vi "new FGGA Serial Data Server & Recordingv4.3_10Hz.vi"(0 "VISA resource name out":refnum<visa-resource-name>, 11 "error IO":errorcluster) -> ()   [LabVIEW 2014]
uses:
  <vilib>/Platform/TimedLoop/XDataNode/timing_clust.ctl
  <vilib>/Platform/TimedLoop/XDataNode/nitl_modes.ctl
  <vilib>/Platform/TimedLoop/XDataNode/wakeup.ctl
  C:/Program Files (x86)/National Instruments/LabVIEW 2014/examples/Data Communication/Network Streams/Simple Network Streams/support/Network Stream Command.ctl
  <vilib>/Utility/error.llb/whitespace.ctl
  <vilib>/Instr/_visa.llb/VISA Flush IO Buffer Mask.ctl
  <vilib>/Instr/_visa.llb/VISA Configure Serial Port (Instr).vi
  <vilib>/Utility/tcp.llb/UDP Multicast Write-Only Open.vi
  <vilib>/platform/TimedLoop/XDataNode/XDataNode.xnode
  <vilib>/Platform/TimedLoop/XDataNode/XDNodeRunTimeDep.lvlib
panel:
  out "ASCII_file_out":string
  out "Unix time":u32
  out "FGGA Pump":bool
  out "Flight Number":string
  out "Stop File Write":bool
  out "Default file name":string
  out "MFC":dbl[](array[numeric])
  out "FGGA restart":bool
  out "V4":bool
  out "V3":bool
  out "V2":bool
  out "V1":bool
  out "error out 2":errorcluster
  out "error out":errorcluster
  in  "MFC_1 SLPM set value":dbl
  out "Value Read":string
  out "status":bool
  in  "VISA resource name":refnum<visa-resource-name>="ASRL3::INSTR"
  in  "timeout (10sec) 2":u32=3000
  in  "Clear Display\nErrors":bool
  out "Data Processing":bool
  out "TCP Binary Packet":string
  out "UDP Time Stamp Offset":i32=1
  out "Data String":string
  out "UDP_ACSII_Out":string
  out "Serial error out":errorcluster
  out "SEPTIC TCP Error Out":errorcluster
  out "TCP packet\nSend To SEPTIC":bool
  out "FISH TCP Error Out":errorcluster
  out "TCP packet\nSend To FISH":bool
  out "UDP_Pack_num":u32
  out "UDP_Out Status":bool
  out "UDP_Out_Error Out":errorcluster
  out "Data Array":string[](array[string])
  out "RAW DATA":string
  in  "stop":bool
  out "Number of times \nRead time out":u32
  out "Loop count":i32
  # "Date"
  # "Time"
  # "CH4_wet_ppm"
  # "1"
  # "H2O_ppm"
  # "CO2_wet_ppm"
  # "CH4_dry_ppm"
  # "CO2_dry_ppm"
  # "cell_pressure_torr"
  # "cell_temp_degC"
  # "ambient(bench)_temp_degC"
  # "RDA_us"
  # "RDB_us"
  # "Fitflag"
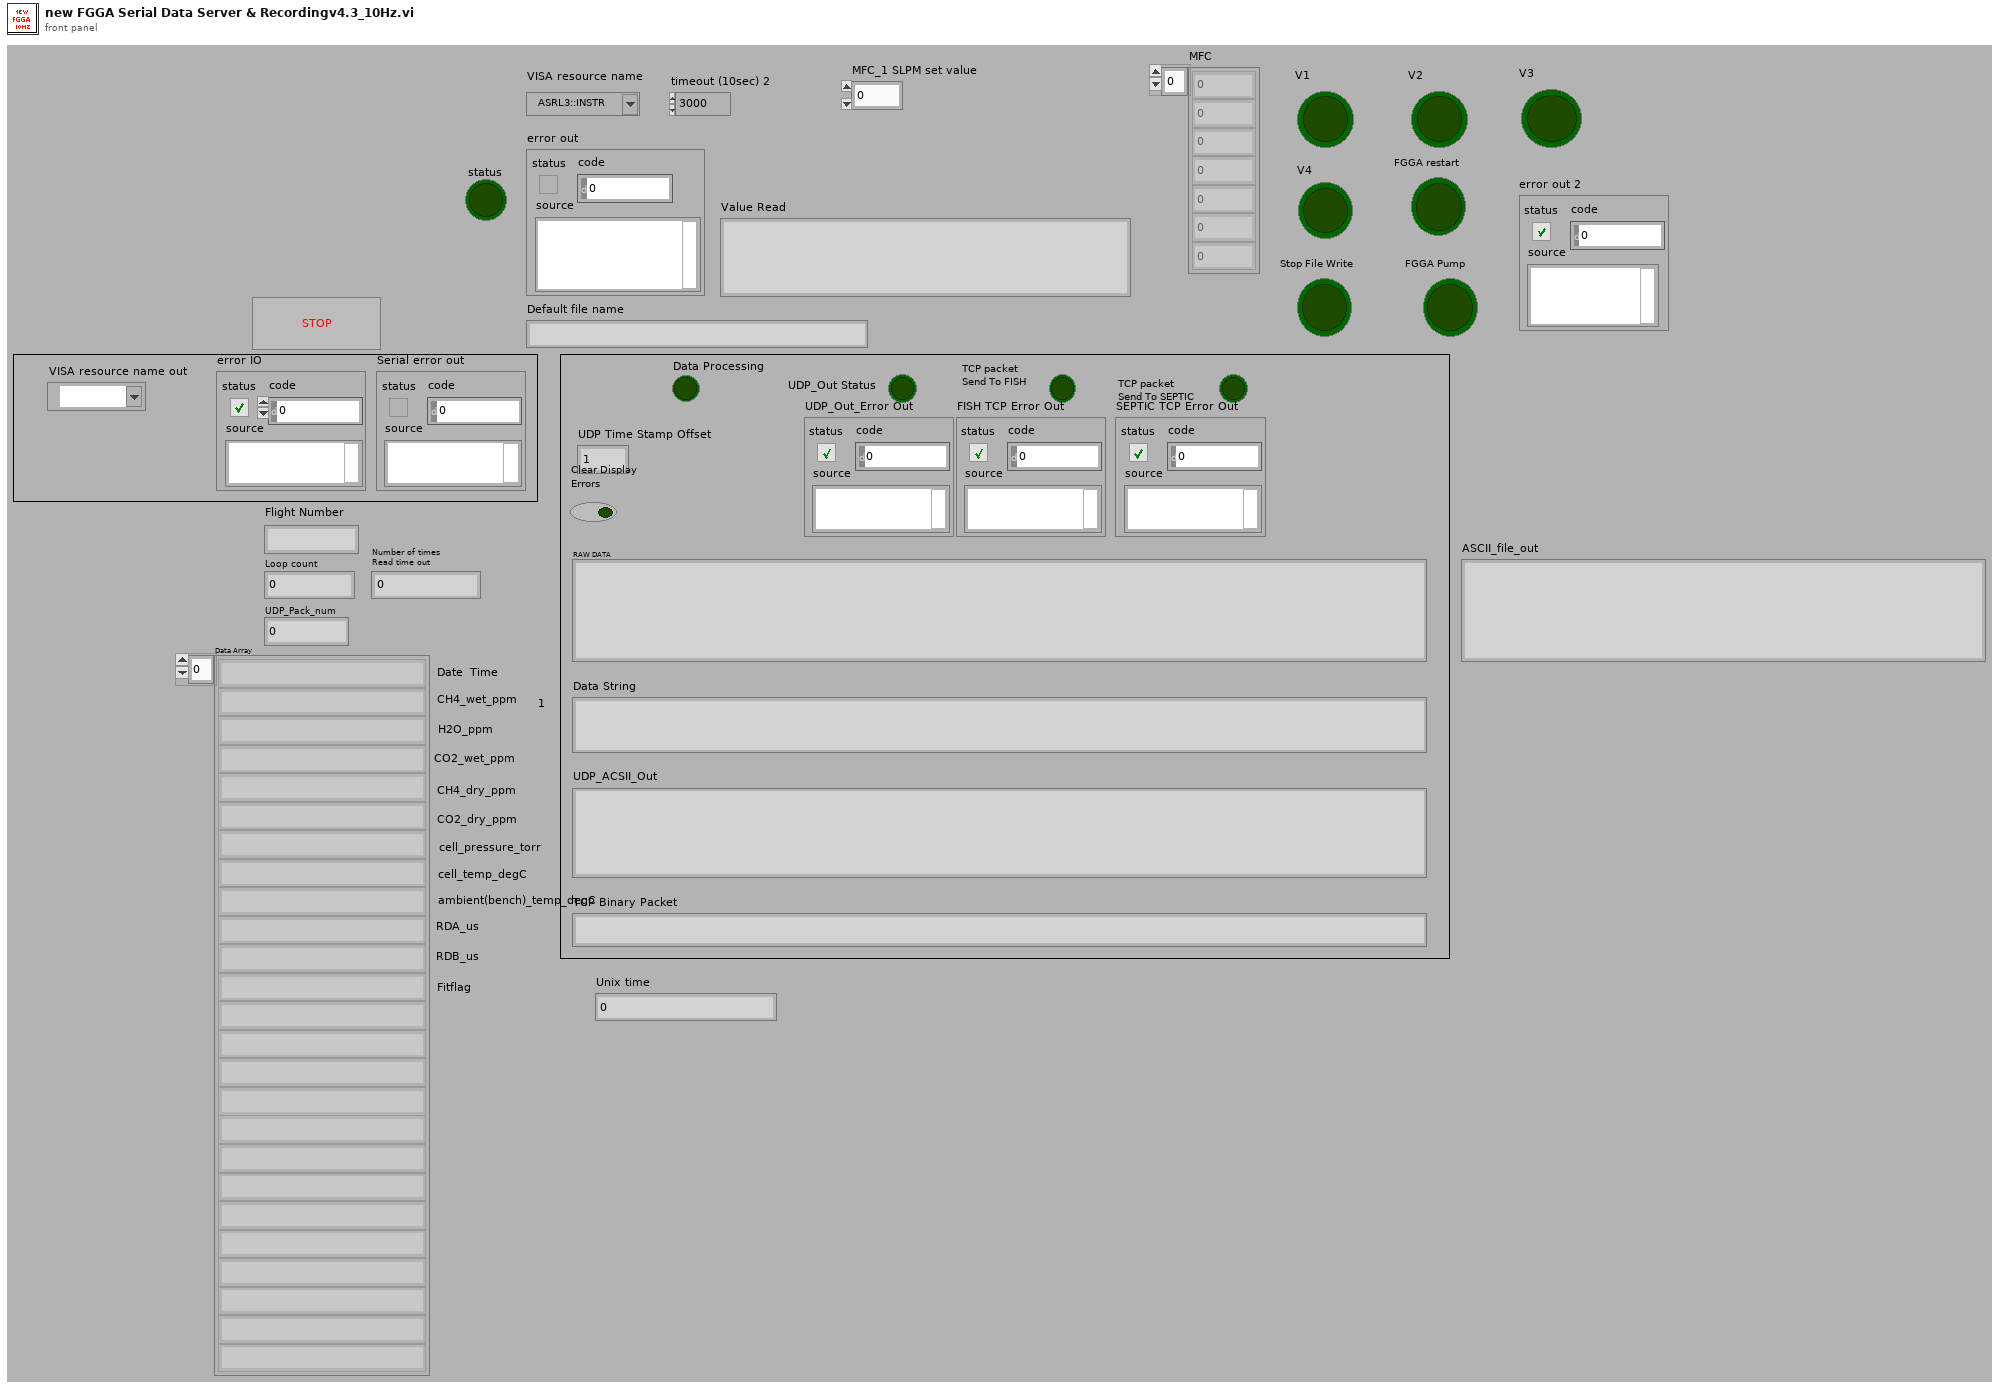
[diagram p1: front panel]
types:
  T1 = typedef "XDNodeRunTimeDep.lvlib/timing_clust.ctl" = cluster{"Expected End [f-1]":u64, "Actual End [f-1]":u64, "Finished Late? [f-1]":bool, "Expected End [i-1]":u64, "Actual End [i-1]":u64, "Finished Late? [i-1]":bool, "Expected Start [i]":u64, "Actual Start [i]":u64, "Expected Start [f]":u64, "Actual Start [f]":u64, "Source Name":string, "Structure Name":string, "Period":i64, "Deadline":i64, "Offset":i64, "Start":i64, "Priority":i32, "Timeout":i32, "Mode":T2, "Wakeup Reason":T3, "Error":errorcluster, "Source Type":string, "Secondary Source Type":string, "Global End Time":u64, "Global Start Time":u64, "Frame Duration":u64, "Iteration Duration":u64, "Assigned CPU":i32, "I/O Scan Engine Mode":u32}
  T2 = typedef "XDNodeRunTimeDep.lvlib/nitl_modes.ctl" = enum32{"No Change", "Process missed periods, maintain original phase", "Discard missed periods, maintain original phase", "Process missed periods, ignore original phase", "Discard missed periods, ignore original phase"}
  T3 = typedef "XDNodeRunTimeDep.lvlib/wakeup.ctl" = enum32{"Normal", "Aborted", "Asynchronous wakeup", "Timing source error", "Timed loop error", "Timeout"}
  T4 = enum16{"open", "replace", "create", "open or create", "replace or create", "replace or create with confirmation"}
  T5 = typedef "Network Stream Command.ctl" = cluster{"Message":string, "Message Data":variant}
  T6 = typedef "whitespace.ctl" = u16
  T7 = typedef "VISA Flush IO Buffer Mask.ctl" = u16
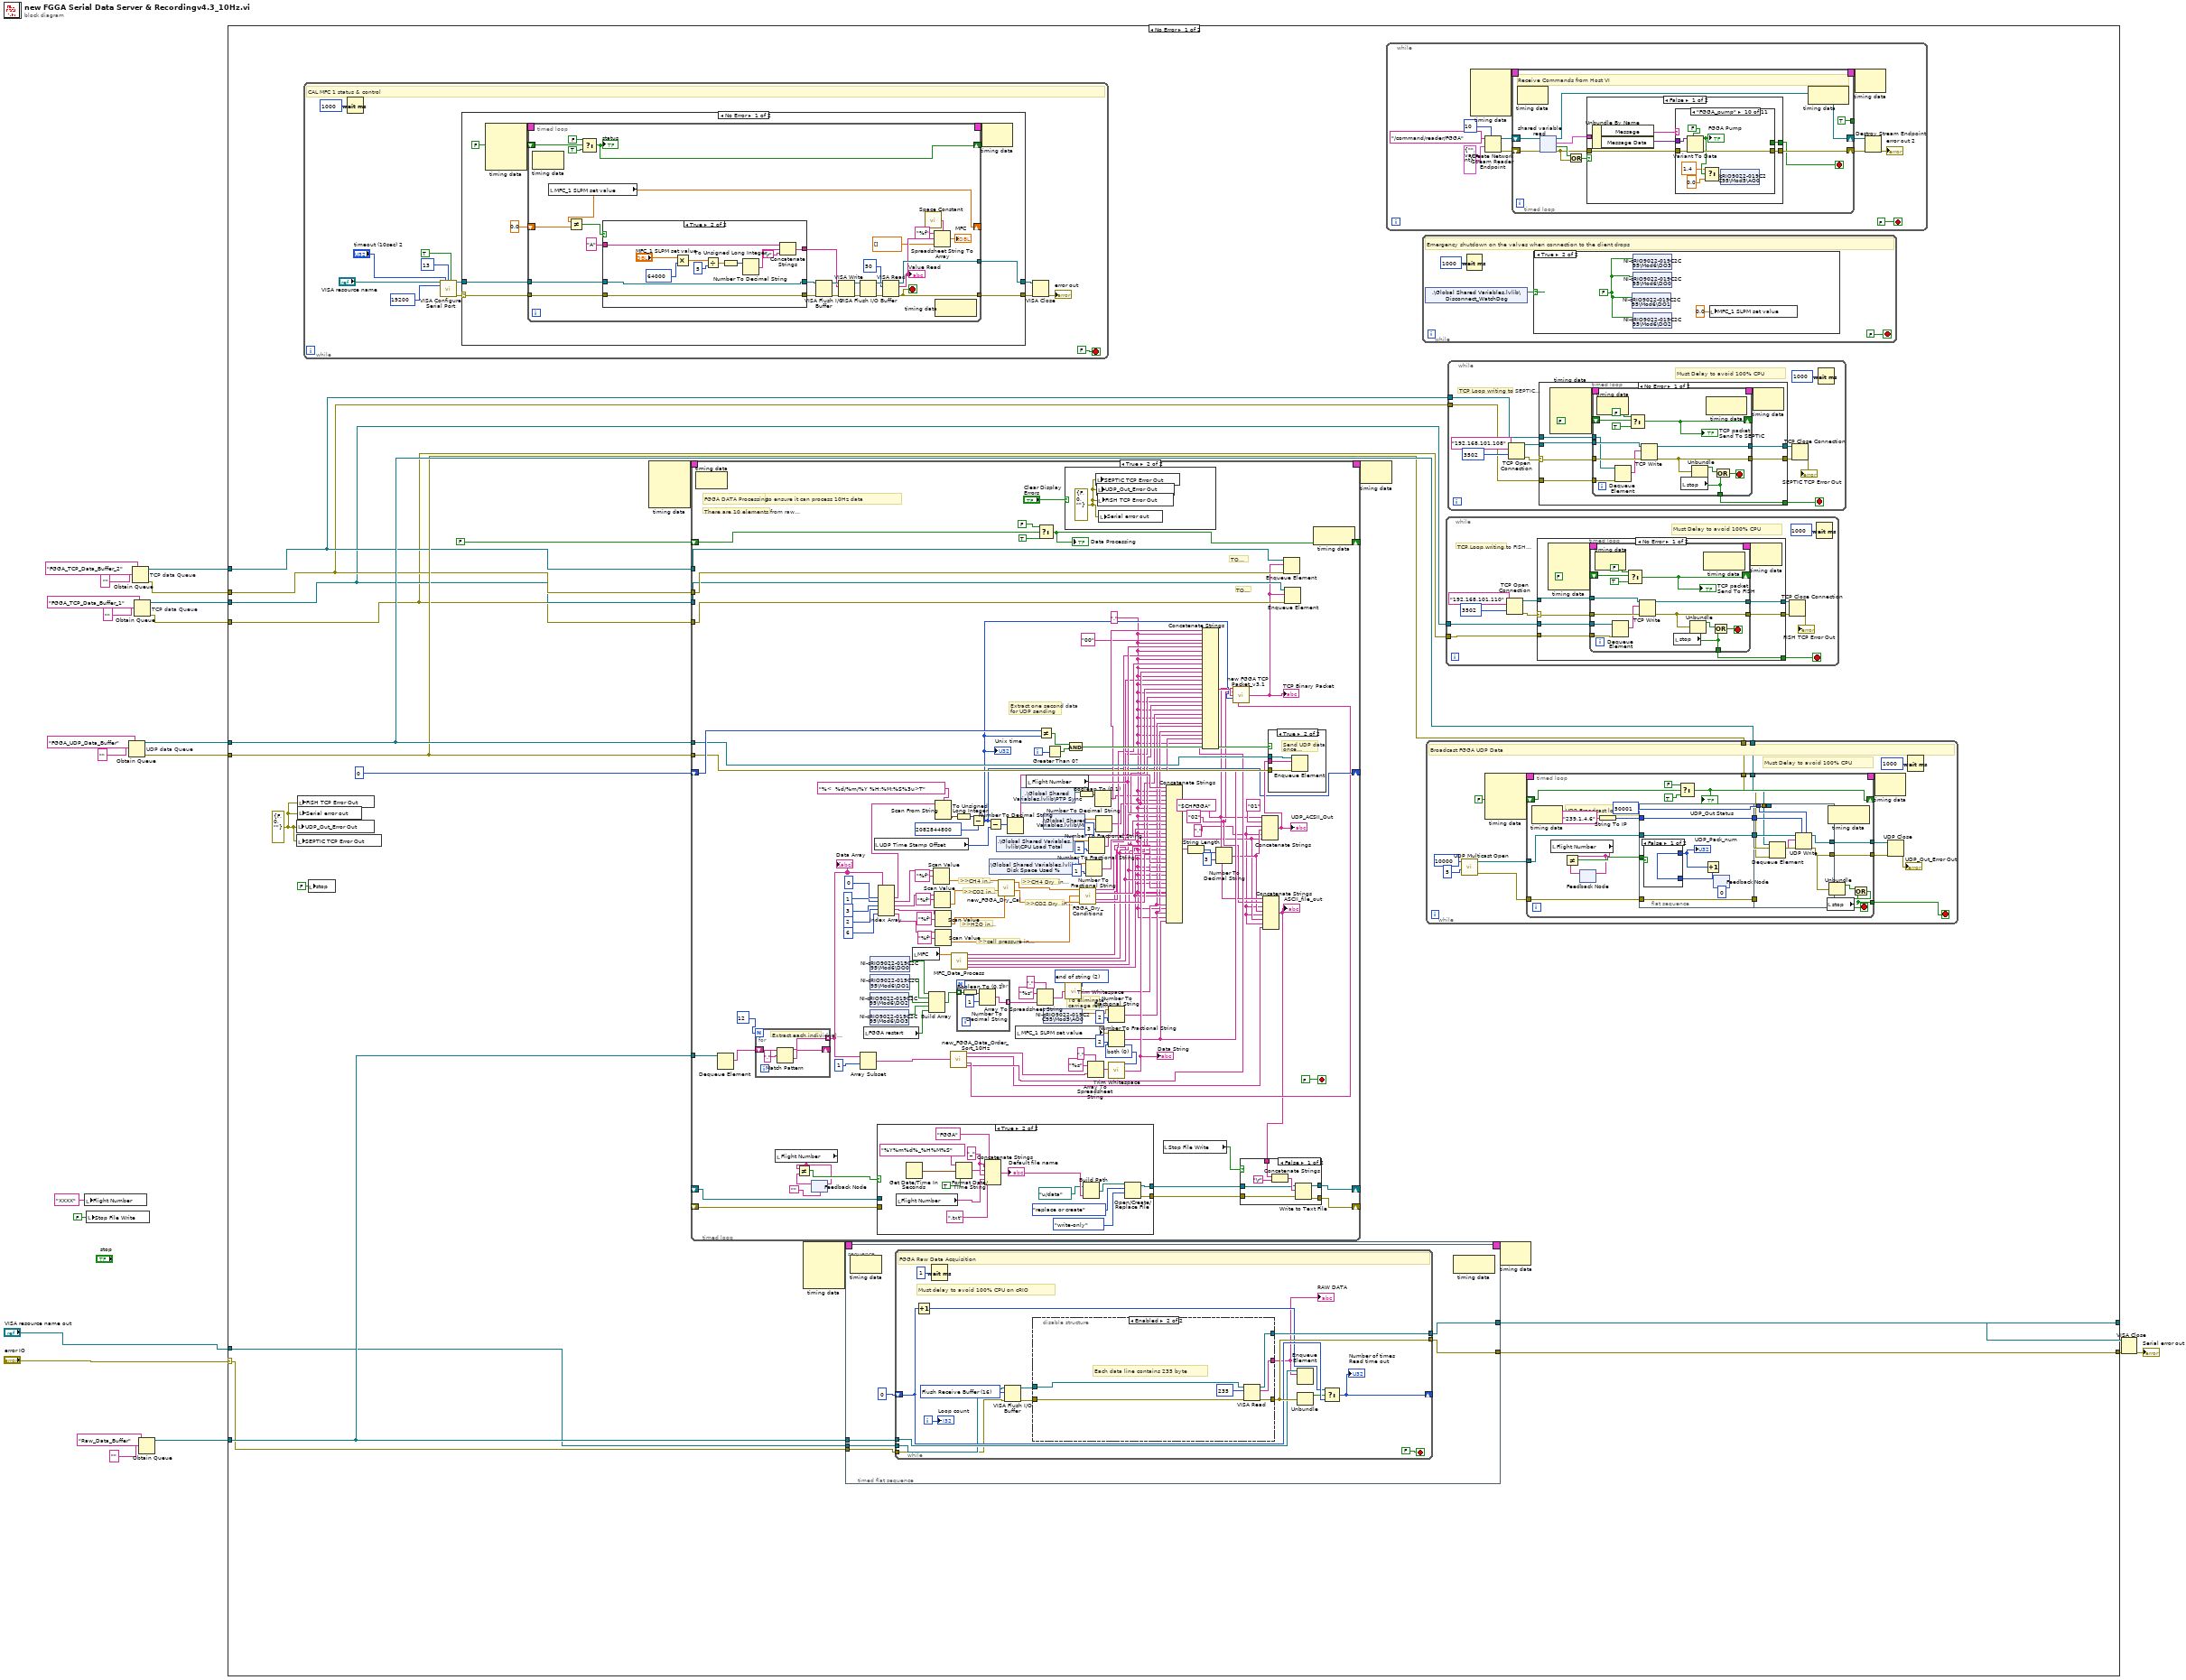
[diagram p0: block diagram]
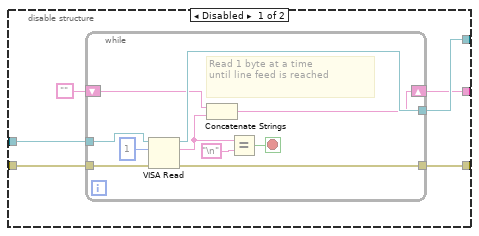
[diagram p2: hidden frame]
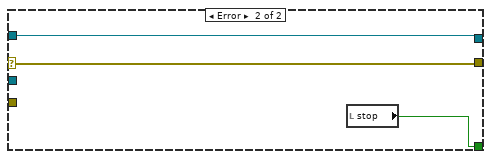
[diagram p3: hidden frame]
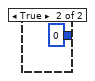
[diagram p4: hidden frame]
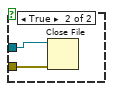
[diagram p6: hidden frame]
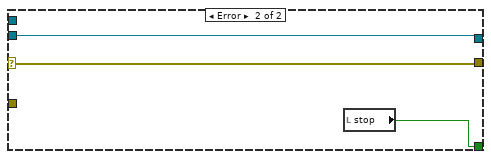
[diagram p9: hidden frame]
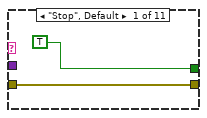
[diagram p11: hidden frame]
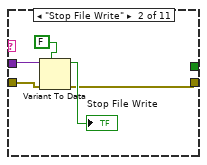
[diagram p12: hidden frame]
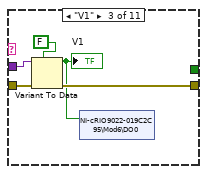
[diagram p13: hidden frame]
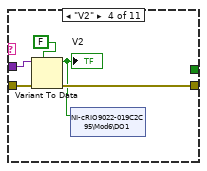
[diagram p14: hidden frame]
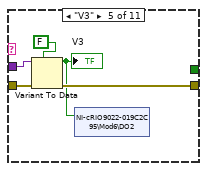
[diagram p15: hidden frame]
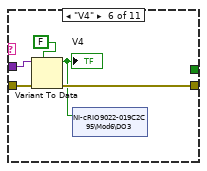
[diagram p16: hidden frame]
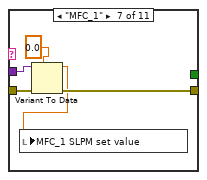
[diagram p17: hidden frame]
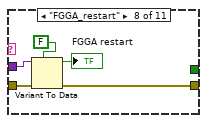
[diagram p18: hidden frame]
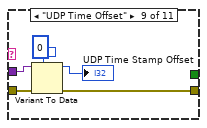
[diagram p19: hidden frame]
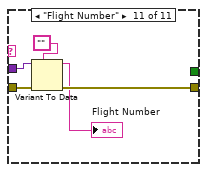
[diagram p20: hidden frame]
diagram:
  n1 = local write "Flight Number"("XXXX" ("Flight Number")) -> ()
  n2 = local write "Stop File Write"(FALSE ("Stop File Write")) -> ()
  n3 = Obtain Queue "UDP data Queue"(name (unnamed)="FGGA_UDP_Data_Buffer", element data type="") -> (queue out=w14:refnum<queue>, error out=w13:errorcluster)  [unwired: 3 in, 1 out]
  n4 = Obtain Queue "TCP data Queue"(name (unnamed)="FGGA_TCP_Data_Buffer_2", element data type="") -> (queue out=w8:refnum<queue>, error out=w7:errorcluster)  [unwired: 3 in, 1 out]
  n5 = Obtain Queue "TCP data Queue"(name (unnamed)="FGGA_TCP_Data_Buffer_1", element data type="") -> (queue out=w6:refnum<queue>, error out=w5:errorcluster)  [unwired: 3 in, 1 out]
  n6 = Obtain Queue(name (unnamed)="Raw_Data_Buffer", element data type="") -> (queue out=w20:refnum<queue>)  [unwired: 3 in, 2 out]
  n7 = case shown="No Error" "error IO" {
    selector: "error IO" -> [w28 w569]
    tunnel: "VISA resource name out" -> [w29 w570]
    tunnel: [w40 w570] -> w17
    tunnel: [w41 w569] -> w18
    tunnel: w20 -> [w39 _]
    tunnel: w14 -> [w37 _]
    tunnel: w13 -> [w36 _]
    tunnel: w8 -> [w35 _]
    tunnel: w7 -> [w34 _]
    tunnel: w6 -> [w33 _]
    tunnel: w5 -> [w32 _]
    frame No Error {
      w25 = errorcluster {"status"=FALSE, "code"=0, "source"=""} ("UDP Error Out")
      n8 = local write "UDP_Out_Error Out"(w25) -> ()
      n9 = local write "SEPTIC TCP Error Out"(w25) -> ()
      n10 = local write "FISH TCP Error Out"(w25) -> ()
      n11 = local write "Serial error out"(w25) -> ()
      n12 = while {
        stop <- FALSE stop-if-true
        # "CAL MFC 1 status & control"
        n13 = Wait (ms)(milliseconds to wait=u32 1000) -> ()  [unwired: 1 out]
        n14 = call-poly "VISA Configure Serial Port"("VISA resource name"="VISA resource name", "timeout (10sec)"="timeout (10sec) 2", "termination char\n(0xA = '\\n' = LF)"=u8 13 ("termination char\n(0xA = '\\n' = LF)"), "Enable Termination\nChar (T)"=TRUE ("Enable Termination\nChar (T)"), "baud rate (9600)"=u32 19200) -> ("VISA resource name out"=w510:refnum<visa-resource-name>, "error out"=w506:errorcluster)  [unwired: 9 in]
        n15 = case shown="No Error" w506 {
          selector: w506 -> [w517 w567]
          tunnel: w510 -> [w518 w568]
          tunnel: [w516 w568] -> w509
          tunnel: [w515 w567] -> w508
          frame No Error {
            n16 = node-c288() -> (w513:T1)  [unwired: 4 in]
            n17 = timed-loop {
              tunnel: w518 -> [w541]
              tunnel: w517 -> [w539]
              tunnel: [w532] -> w516
              tunnel: [w527] -> w515
              shift-right: [w528] -> _
              shift-left: FALSE -> [w531]
              timing: w513 -> [_]
              timing-out: [_] -> w512
              shift-right: [w519] -> _
              shift-left: 0.0 -> [w521]
              stop <- w527 stop-if-true
              n18 = node-c288() -> ()  [unwired: 1 in, 1 out]
              n19 = local read "MFC_1 SLPM set value"() -> (w519:dbl)
              n20 = Not Equal?(x=w519, y=w521) -> (x != y?=w520:bool)
              n21 = Select(t=FALSE, s=w531, f=TRUE) -> (s? t:f=w528:bool)
              "status" <- w528
              n22 = case shown="True" w520 {
                tunnel: w541 -> [w549 w564]
                tunnel: [w549 w564] -> w540
                tunnel: w539 -> [w548 w563]
                tunnel: [w548 w563] -> w538
                tunnel: "A" -> [w552 w556]
                tunnel: [w550 w553] -> w536
                frame False {
                  n23 = Concatenate Strings(w552, "\r") -> (w550:string)
                }
                frame True {
                  n24 = Multiply(x="MFC_1 SLPM set value", y=u32 64000) -> (x*y=w560:dbl)
                  n25 = Divide(x=w560, y=u32 5) -> (x/y=w558:dbl)
                  n26 = To Unsigned Long Integer(number=w558) -> (unsigned 32bit integer=w557:u32)
                  n27 = Number To Decimal String(number=w557) -> (decimal integer string=w555:string)  [unwired: 1 in]
                  n28 = Concatenate Strings(w556, w555, "\r") -> (w553:string)
                }
              }
              n29 = VISA Flush I/O Buffer(VISA resource name=w540, error in (no error)=w538) -> (VISA resource name out=w543:refnum<visa-resource-name>, error out=w542:errorcluster)  [unwired: 1 in]
              n30 = VISA Write(VISA resource name=w543, write buffer=w536, error in (no error)=w542) -> (VISA resource name out=w535:refnum<visa-resource-name>, error out=w534:errorcluster)  [unwired: 1 out]
              n31 = VISA Flush I/O Buffer(VISA resource name=w535, error in (no error)=w534) -> (VISA resource name out=w545:refnum<visa-resource-name>, error out=w544:errorcluster)  [unwired: 1 in]
              n32 = VISA Read(VISA resource name=w545, byte count=u32 50, error in (no error)=w544) -> (VISA resource name out=w532:refnum<visa-resource-name>, read buffer=w526:string, error out=w527:errorcluster)  [unwired: 1 out]
              "Value Read" <- w526
              n33 = call <vilib>:"Space Constant.vi"() -> ("String"=w525:string)
              n34 = Spreadsheet String To Array(delimiter (Tab)=w525, format string="%f", spreadsheet string=w526, array type (2D Dbl)=dbl[] []) -> (array=→"MFC":dbl[])
              n35 = node-c288() -> ()  [unwired: 1 in, 1 out]
            }
            n36 = node-c288(w512) -> ()  [unwired: 1 out]
          }
          frame Error {
          }
        }
        n37 = VISA Close(VISA resource name=w509, error in (no error)=w508) -> (error out=→"error out":errorcluster)
      }
      n38 = local write "stop"(FALSE ("stop")) -> ()
      n39 = node-c288() -> (w27:T1)  [unwired: 4 in]
      n40 = timed-loop {
        timing: w27 -> [_]
        timing-out: [_] -> w26
        tunnel: w39 -> [w321]
        tunnel: w37 -> [w289]
        tunnel: w36 -> [w288]
        shift-right: [w216] -> _
        shift-left: u32 0 -> [w292]
        tunnel: w35 -> [w287]
        tunnel: w34 -> [w286]
        tunnel: w33 -> [w285]
        tunnel: w32 -> [w284]
        shift-right: [w280] -> _
        shift-left: FALSE -> [w283]
        shift-right: [w269] -> _
        shift-left: _ -> [w261]
        shift-right: [w259] -> _
        shift-left: _ -> [w260]
        i -> [w291]
        stop <- FALSE stop-if-true
        w233 = T6 2 items=["both", "start of string", "end of string"] ("location (both)")
        w209 = ","
        w310 = T6 0 items=["both", "start of string", "end of string"] ("location (both)")
        w197 = ","
        w201 = "02"
        w202 = "$CHFGGA"
        # "To eliminate\ncarriage return"
        # ">>cell pressure in torr>>"
        # "There are 10 elements from raw packet"
        # "TO SEPTIC"
        # "TO FISH"
        # "Extract one second data\nfor UDP sending"
        # ">>CO2 Dry  in ppm>>"
        # ">>CH4 Dry  in ppb>>"
        # ">>H2O in ppm>>"
        # ">>CO2 in ppm>>"
        # ">>CH4 in ppm>>"
        # "Loop Time is 50msec to ensure it can process 10Hz data"
        # "FGGA DATA Processing"
        n41 = node-c288() -> ()  [unwired: 1 in, 1 out]
        n42 = Dequeue Element(queue=w321) -> (element=w279:string)  [unwired: 2 in, 3 out]
        n43 = for {
          N: 12 -> [_]
          shift-right: [w358] -> _
          shift-left: w279 -> [w356]
          tunnel: [w357] -> w315 mode=indexing
          # "Extract each individual param"
          n44 = Match Pattern(string=w356, regular expression=",") -> (before substring=w357:string, after substring=w358:string)  [unwired: 1 in, 2 out]
        }
        "Data Array" <- w315
        n45 = local read "Flight Number"() -> (w258:string)
        n46 = feedback #1("" ("Flight Number")) -> (w266:string)
        n47 = Not Equal?(x=w258, y=w266) -> (x != y?=w264:bool)
        n48 = feedback-in #1(w258) -> ()
        n49 = Array Subset(array=w315, index=1) -> (w207:string[])  [unwired: 1 in]
        n50 = local read "FGGA restart"() -> (w243:bool)
        n51 = shared-variable "NI-cRIO9022-019C2C95\\Mod6\\DO2"() -> (w249:bool)  [unwired: 1 in, 1 out]
        n52 = shared-variable "NI-cRIO9022-019C2C95\\Mod6\\DO3"() -> (w248:bool)  [unwired: 1 in, 1 out]
        n53 = shared-variable "NI-cRIO9022-019C2C95\\Mod6\\DO0"() -> (w251:bool)  [unwired: 1 in, 1 out]
        n54 = shared-variable "NI-cRIO9022-019C2C95\\Mod6\\DO1"() -> (w250:bool)  [unwired: 1 in, 1 out]
        n55 = local read "UDP Time Stamp Offset"() -> (w232:i32)
        n56 = case shown="True" w264 {
          tunnel: [w327 w329] -> w263
          tunnel: [w326 w328] -> w262
          tunnel: w261 -> [w327 _]
          tunnel: w260 -> [w326 _]
          frame False {
          }
          frame True {
            w335 = "_" ("string")
            n57 = local read "Flight Number"() -> (w342:string)
            n58 = Get Date/Time In Seconds() -> (seconds since 1Jan1904=w330:timestamp)
            n59 = Format Date/Time String(time format string (%c)="%Y%m%d%_%H%M%S", seconds (now)=w330, UTC format=TRUE) -> (date/time string=w332:string)
            n60 = Concatenate Strings("FGGA" ("string"), w335, w332, w335, w342, ".txt" ("string")) -> (w337:string)
            "Default file name" <- w337
            n61 = Build Path(base path=path "u:/data", name or relative path=w337) -> (appended path=w341:path)
            n62 = Open/Create/Replace File(file path (use dialog)=w341, operation (0:open)=T4."replace or create", access (0:read/write)=enum16{"read/write", "read-only", "write-only"}."write-only") -> (refnum out=w329:refnum<file>, error out=w328:errorcluster)  [unwired: 3 in, 1 out]
          }
        }
        n63 = Index Array(array=w315, index #1=0 ("index"), index #2=1 ("index"), index #3=3 ("index"), index #4=2 ("index"), index #5=6 ("index")) -> (element #1=w210:string, element #2=w215:string, element #3=w214:string, element #4=w213:string, element #5=w212:string)
        n64 = local read "MFC"() -> (w270:dbl[])
        n65 = Build Array(w251, w250, w249, w248, w243) -> (w247:bool[])
        n66 = Scan Value(string=w215, format string="%f") -> (value=w301:dbl)  [unwired: 1 in, 1 out]
        n67 = Scan Value(string=w214, format string="%f") -> (value=w300:dbl)  [unwired: 1 in, 1 out]
        n68 = Scan From String(format string="%<  %d/%m/%Y %H:%M:%S%3u>T", input string=w210) -> (output 1=w297:timestamp)  [unwired: 3 in, 3 out]
        n69 = Scan Value(string=w213, format string="%f") -> (value=w271:dbl)  [unwired: 1 in, 1 out]
        n70 = Scan Value(string=w212, format string="%f") -> (value=w272:dbl)  [unwired: 1 in, 1 out]
        n71 = call "new_FGGA_Data_Order_Sort_10Hz.vi"("Data In"=w207) -> ("UDP Data Out"=w206:string[], "ASCII Ambient(bench)_temp"=w196:string, "TCP Data Out"=w205:string[], "TCP Ambient(bench)_temp"=w204:string)  [unwired: 11 in]
        n72 = call "MFC_Data_Process.vi"("MFC"=w270) -> ("MFC Absolute Pressure"=w227:string, "MFC Temperature"=w226:string, "MFC Volumetric Flow"=w225:string, "MFC Mass Flow"=w224:string, "MFC Set Point"=w223:string)  [unwired: 10 in]
        n73 = To Unsigned Long Integer(number=w297) -> (unsigned 32bit integer=w298:u32)
        n74 = for {
          tunnel: w247 -> [w324] mode=indexing
          tunnel: [w323] -> w244 mode=indexing
          n75 = Boolean To (0,1)(Boolean=w324) -> (0, 1=w325:i16)
          n76 = Number To Decimal String(number=w325, width (-)=i16 1) -> (decimal integer string=w323:string)
        }
        n77 = Subtract(x=w298, y=u32 2082844800) -> (x-y=w216:u32)
        "Unix time" <- w216
        n78 = Subtract(x=w216, y=w232) -> (x-y=w295:u32)
        n79 = shared-variable ".\\Global Shared Variables.lvlib\\Disk Space Used %"() -> (w236:dbl)  [unwired: 1 in, 1 out]
        n80 = shared-variable ".\\Global Shared Variables.lvlib\\CPU Load Total"() -> (w257:dbl)  [unwired: 1 in, 1 out]
        n81 = call "new_FGGA_Dry_Cal.vi"("H2O"=w271, "CO2_Wet"=w300, "CH4_Wet"=w301) -> ("CO2_Dry"=w274:dbl, "CH4_Dry"=w276:dbl)  [unwired: 7 in]
        n82 = Number To Decimal String(number=w295) -> (decimal integer string=w296:string)  [unwired: 1 in]
        n83 = local read "MFC_1 SLPM set value"() -> (w239:dbl)
        n84 = shared-variable ".\\Global Shared Variables.lvlib\\PTP Sync"() -> (w252:bool)  [unwired: 1 in, 1 out]
        n85 = local read "Flight Number"() -> (w231:string)
        n86 = Array To Spreadsheet String(delimiter (Tab)=",", array=w244, 3:"%s" ("format string")) -> (spreadsheet string=w234:string)
        n87 = Select(t=FALSE, s=w283, f=TRUE) -> (s? t:f=w280:bool)
        "Data Processing" <- w280
        n88 = Not Equal?(x=w292, y=w216) -> (x != y?=w293:bool)
        n89 = shared-variable ".\\Global Shared Variables.lvlib\\MFM"() -> (w255:dbl)  [unwired: 1 in, 1 out]
        n90 = shared-variable "NI-cRIO9022-019C2C95\\Mod5\\AO0"() -> (w241:dbl)  [unwired: 1 in, 1 out]
        n91 = Greater Than 0?(x=w291) -> (x > 0?=w294:bool)
        n92 = case shown="True" "Clear Display\nErrors" {
          frame False {
          }
          frame True {
            w352 = errorcluster {"status"=FALSE, "code"=0, "source"=""} ("UDP Error Out")
            n93 = local write "SEPTIC TCP Error Out"(w352) -> ()
            n94 = local write "UDP_Out_Error Out"(w352) -> ()
            n95 = local write "FISH TCP Error Out"(w352) -> ()
            n96 = local write "Serial error out"(w352) -> ()
          }
        }
        n97 = call <vilib>:"Trim Whitespace.vi"("string"=w234, "location (both)"=w233) -> ("trimmed string"=w222:string)
        n98 = Compound Arithmetic op=AND(w293, w294) -> (w290:bool)
        n99 = Boolean To (0,1)(Boolean=w252) -> (0, 1=w253:i16)
        n100 = call "FGGA_Dry_Conditions.vi"("CH4_Dry"=w276, "Pressure"=w272, "CO2_Dry"=w274) -> ("CH4_Dry_TCP"=w230:string, "CH4_Dry_UDP"=w278:string, "CO2_Dry_TCP"=w229:string, "CO2_Dry_UDP"=w277:string)  [unwired: 9 in]
        n101 = Number To Fractional String(number=w236, precision (6)=i16 1) -> (F-format string=w235:string)  [unwired: 2 in]
        n102 = Array To Spreadsheet String(delimiter (Tab)=",", array=w206, 3:"%s" ("format string")) -> (spreadsheet string=w309:string)
        n103 = Number To Fractional String(number=w257, precision (6)=i16 2) -> (F-format string=w238:string)  [unwired: 2 in]
        n104 = Number To Decimal String(number=w253) -> (decimal integer string=w218:string)  [unwired: 1 in]
        n105 = Number To Fractional String(number=w255, precision (6)=i16 3) -> (F-format string=w228:string)  [unwired: 2 in]
        n106 = Number To Fractional String(number=w241, precision (6)=i16 2) -> (F-format string=w221:string)  [unwired: 2 in]
        n107 = Number To Fractional String(number=w239, precision (6)=i16 2) -> (F-format string=w220:string)  [unwired: 2 in]
        n108 = call <vilib>:"Trim Whitespace.vi"("string"=w309, "location (both)"=w310) -> ("trimmed string"=w308:string)
        "Data String" <- w308
        n109 = local read "Stop File Write"() -> (w267:bool)
        n110 = Concatenate Strings(w296, w209, w218, w209, w228, w209, w231, w209, w238, w209, w235, w209, w308, w209, w278, w209, w277, w209, w227, w209, w226, w209, w225, w209, w224, w209, w223, w209, w222, w209, w221, w209, w220) -> (w199:string)
        n111 = String Length(string=w199) -> (length=w318:i32)
        n112 = Concatenate Strings(w218, w209, "00", w209, w231, w209, w230, w209, w229, w209, w228, w209, w227, w209, w226, w209, w225, w209, w224, w209, w223, w209, w222, w209, w221, w209, w220, w209, w204) -> (w219:string)
        n113 = Number To Decimal String(number=w318, width (-)=i16 3) -> (decimal integer string=w200:string)
        n114 = call "new FGGA TCP Packet_v3.1.vi"("ID"=w202, "Version"=w201, "TCP Packet In"=w219, "utc_time"=w216, "Data Array"=w205) -> ("TCP Binary Packet"=w208:string)  [unwired: 10 in]
        "TCP Binary Packet" <- w208
        n115 = Concatenate Strings(w202, "01", w197, w200, w197, w199) -> (w268:string)
        "UDP_ACSII_Out" <- w268
        n116 = Concatenate Strings(w202, w201, w197, w200, w197, w199, w197, w196) -> (w198:string)
        "ASCII_file_out" <- w198
        n117 = case shown="False" w267 {
          tunnel: w198 -> [w349 _]
          tunnel: [w346 _] -> w269
          tunnel: w263 -> [w345 w351]
          tunnel: w262 -> [w344 w350]
          tunnel: [w343 _] -> w259
          frame False {
            n118 = Concatenate Strings(w349, "\r") -> (w347:string)
            n119 = Write to Text File(file (use dialog)=w345, text=w347, error in=w344) -> (refnum out=w346:refnum<file>, error out=w343:errorcluster)  [unwired: 2 out]
          }
          frame True {
            n120 = Close File(refnum=w351, error in=w350) -> ()  [unwired: 2 out]
          }
        }
        n121 = case shown="True" w290 {
          tunnel: w268 -> [_ w355]
          tunnel: w289 -> [_ w354]
          tunnel: w288 -> [_ w353]
          frame False {
          }
          frame True {
            # "Send UDP data once\na second"
            n122 = Enqueue Element(queue=w354, element=w355, error in (no error)=w353) -> ()  [unwired: 1 in, 3 out]
          }
        }
        n123 = Enqueue Element(queue=w287, element=w208, error in (no error)=w286) -> ()  [unwired: 1 in, 3 out]
        n124 = Enqueue Element(queue=w285, element=w208, error in (no error)=w284) -> ()  [unwired: 1 in, 3 out]
        n125 = node-c288() -> ()  [unwired: 1 in, 1 out]
      }
      n126 = node-c288() -> (w24:T1)  [unwired: 4 in]
      n127 = timed-sequence {
        timing: w24 -> [_]
        timing-out: [_] -> w23
        tunnel: [w46] -> w41
        tunnel: [w45] -> w40
        tunnel: w39 -> [w44]
        tunnel: w29 -> [w43]
        tunnel: w28 -> [w42]
        n128 = timed-flat-sequence {
          tunnel: [w52] -> w46
          tunnel: [w51] -> w45
          tunnel: w44 -> [w50]
          tunnel: w43 -> [w49]
          tunnel: w42 -> [w48]
          n129 = node-c288() -> ()  [unwired: 1 in, 1 out]
          n130 = while {
            tunnel: w49 -> [w59]
            tunnel: w48 -> [w58]
            tunnel: [w70] -> w52
            shift-right: [w66] -> _
            shift-left: u32 0 -> [w67]
            tunnel: [w69] -> w51
            tunnel: w50 -> [w64]
            i -> [w68]
            stop <- FALSE stop-if-true
            w55 = T7 16 items=["Flush Receive Buffer"=16, "Write Transmit Buffer to Device"=32, "Flush Receive Buffer (No I/O)"=64, "Flush Transmit Buffer"=128] ("Mask")
            # "Must delay to avoid 100% CPU on cRIO"
            # "FGGA Raw Data Acquisition"
            n131 = Increment(x=w67) -> (x+1=w65:u32)
            n132 = Wait (ms)(milliseconds to wait=u32 1) -> ()  [unwired: 1 out]
            n133 = VISA Flush I/O Buffer(VISA resource name=w59, mask (16)=w55, error in (no error)=w58) -> (VISA resource name out=w56:refnum<visa-resource-name>, error out=w57:errorcluster)
            n134 = disable-structure shown="Enabled" {
              disable-tunnel: [w76 w90] -> w70
              disable-tunnel: [w75 w89] -> w69
              disable-tunnel: [w74 w88] -> w61
              disable-tunnel: w57 -> [w73 w91]
              disable-tunnel: w56 -> [w72 w92]
              frame Disabled {
                n135 = while {
                  tunnel: [w86] -> w75
                  tunnel: [w85] -> w76
                  tunnel: w72 -> [w84]
                  tunnel: w73 -> [w83]
                  shift-right: [w81] -> w74
                  shift-left: "" -> [w82]
                  stop <- w78 stop-if-true
                  # "Read 1 byte at a time \nuntil line feed is reached"
                  n136 = VISA Read(VISA resource name=w84, byte count=u32 1, error in (no error)=w83) -> (VISA resource name out=w86:refnum<visa-resource-name>, read buffer=w80:string, error out=w85:errorcluster)  [unwired: 1 out]
                  n137 = Concatenate Strings(w82, w80) -> (w81:string)
                  n138 = Equal?(x=w80, y="\n") -> (x = y?=w78:bool)
                }
              }
              frame Enabled {
                # "Each data line contains 235 byte"
                n139 = VISA Read(VISA resource name=w92, byte count=u32 235, error in (no error)=w91) -> (VISA resource name out=w89:refnum<visa-resource-name>, read buffer=w88:string, error out=w90:errorcluster)  [unwired: 1 out]
              }
            }
            "RAW DATA" <- w61
            n140 = Enqueue Element(queue=w64, element=w61) -> ()  [unwired: 2 in, 3 out]
            n141 = Unbundle(w70) -> ("status"=w63:bool)  [unwired: 2 out]
            n142 = Select(t=w65, s=w63, f=w67) -> (s? t:f=w66:u32)
            "Number of times \nRead time out" <- w66
            "Loop count" <- w68
          }
          n143 = node-c288() -> ()  [unwired: 1 in, 1 out]
        }
      }
      n144 = node-c288(w26) -> ()  [unwired: 1 out]
      n145 = while {
        stop <- FALSE stop-if-true
        n146 = node-c288() -> (w412:T1)  [unwired: 4 in]
        n147 = Create Network Stream Reader Endpoint(7:10 ("reader buffer size"), 9:T5 {"Message"="", "Message Data"=variant} ("Message Cluster"), 11:"/command/reader/FGGA" ("reader url")) -> (0:w417:errorcluster, 3:w418:refnum<k21>)  [unwired: 4 in]
        n148 = timed-loop "Host->Target Command Reader" {
          shift-right: [w428] -> w415
          shift-left: w417 -> [w431]
          shift-right: [w429] -> w414
          shift-left: w418 -> [w430]
          tunnel: [TRUE] -> _
          timing: w412 -> [_]
          timing-out: [_] -> w411
          stop <- w422 stop-if-true
          # "Receive Commands from Host VI"
          n149 = node-c288() -> ()  [unwired: 1 in, 1 out]
          n150 = shared-variable-read(w430, w431) -> (w429:refnum<k21>, w424:errorcluster, w426:bool, w427:T5)  [unwired: 1 in]
          n151 = Or(x=w426, y=w424) -> (x .or. y?=w425:bool)
          n152 = case shown="False" w425 {
            selector: w425 -> [_ w495]
            tunnel: w424 -> [w439 w496]
            tunnel: [w438 w496] -> w428
            tunnel: w427 -> [w436 _]
            tunnel: [w437 w495] -> w422
            frame False {
              n153 = Unbundle By Name(w436) -> ("Message"=w435:string, "Message Data"=w434:variant)
              n154 = case shown="\"FGGA_pump\"" w435 {
                tunnel: w439 -> [w441 w446 w451 w456 w461 w466 w471 w476 w481 w489 w494]
                tunnel: [w441 w442 w450 w455 w460 w465 w470 w475 w480 w488 w493] -> w438
                tunnel: w434 -> [_ w445 w449 w454 w459 w464 w469 w474 w479 w487 w492]
                tunnel: [TRUE _ _ _ _ _ _ _ _ _ _] -> w437
                frame "Stop", Default {
                }
                frame "Stop File Write" {
                  n155 = Variant To Data(error in=w446, type=FALSE, Variant=w445) -> (data=→"Stop File Write":bool, error out=w442:errorcluster)
                }
                frame "V1" {
                  n156 = Variant To Data(error in=w451, type=FALSE, Variant=w449) -> (data=w447:bool, error out=w450:errorcluster)
                  "V1" <- w447
                  n157 = shared-variable "NI-cRIO9022-019C2C95\\Mod6\\DO0"(w447) -> ()  [unwired: 1 in, 1 out]
                }
                frame "V2" {
                  n158 = Variant To Data(error in=w456, type=FALSE, Variant=w454) -> (data=w452:bool, error out=w455:errorcluster)
                  "V2" <- w452
                  n159 = shared-variable "NI-cRIO9022-019C2C95\\Mod6\\DO1"(w452) -> ()  [unwired: 1 in, 1 out]
                }
                frame "V3" {
                  n160 = Variant To Data(error in=w461, type=FALSE, Variant=w459) -> (data=w457:bool, error out=w460:errorcluster)
                  "V3" <- w457
                  n161 = shared-variable "NI-cRIO9022-019C2C95\\Mod6\\DO2"(w457) -> ()  [unwired: 1 in, 1 out]
                }
                frame "V4" {
                  n162 = Variant To Data(error in=w466, type=FALSE, Variant=w464) -> (data=w462:bool, error out=w465:errorcluster)
                  "V4" <- w462
                  n163 = shared-variable "NI-cRIO9022-019C2C95\\Mod6\\DO3"(w462) -> ()  [unwired: 1 in, 1 out]
                }
                frame "MFC_1" {
                  n164 = Variant To Data(error in=w471, type=0.0, Variant=w469) -> (data=w467:dbl, error out=w470:errorcluster)
                  n165 = local write "MFC_1 SLPM set value"(w467) -> ()
                }
                frame "FGGA_restart" {
                  n166 = Variant To Data(error in=w476, type=FALSE, Variant=w474) -> (data=→"FGGA restart":bool, error out=w475:errorcluster)
                }
                frame "UDP Time Offset" {
                  n167 = Variant To Data(error in=w481, type=0, Variant=w479) -> (data=→"UDP Time Stamp Offset":i32, error out=w480:errorcluster)
                }
                frame "FGGA_pump" {
                  n168 = Variant To Data(error in=w489, type=FALSE, Variant=w487) -> (data=w484:bool, error out=w488:errorcluster)
                  "FGGA Pump" <- w484
                  n169 = Select(t=1.4 ("f"), s=w484, f=0.0 ("t")) -> (s? t:f=w485:dbl)
                  n170 = shared-variable "NI-cRIO9022-019C2C95\\Mod5\\AO0"(w485) -> ()  [unwired: 1 in, 1 out]
                }
                frame "Flight Number" {
                  n171 = Variant To Data(error in=w494, type="", Variant=w492) -> (data=→"Flight Number":string, error out=w493:errorcluster)
                }
              }
            }
            frame True {
            }
          }
          n172 = node-c288() -> ()  [unwired: 1 in, 1 out]
        }
        n173 = node-c288(w411) -> ()  [unwired: 1 out]
        n174 = Destroy Stream Endpoint(8:w415, 11:w414) -> (0:→"error out 2":errorcluster)
      }
      n175 = while {
        stop <- FALSE stop-if-true
        # "Emergency shutdown on the valves when connection to the client drops"
        n176 = shared-variable ".\\Global Shared Variables.lvlib\\Disconnect_WatchDog"() -> (w406:bool)  [unwired: 1 in, 1 out]
        n177 = Wait (ms)(milliseconds to wait=u32 1000) -> ()  [unwired: 1 out]
        n178 = case shown="True" w406 {
          frame False {
          }
          frame True {
            w410 = FALSE
            n179 = shared-variable "NI-cRIO9022-019C2C95\\Mod6\\DO1"(w410) -> ()  [unwired: 1 in, 1 out]
            n180 = shared-variable "NI-cRIO9022-019C2C95\\Mod6\\DO3"(w410) -> ()  [unwired: 1 in, 1 out]
            n181 = shared-variable "NI-cRIO9022-019C2C95\\Mod6\\DO0"(w410) -> ()  [unwired: 1 in, 1 out]
            n182 = shared-variable "NI-cRIO9022-019C2C95\\Mod6\\DO2"(w410) -> ()  [unwired: 1 in, 1 out]
            n183 = local write "MFC_1 SLPM set value"(0.0 ("MFC_1 SLPM set value")) -> ()
          }
        }
      }
      n184 = while {
        tunnel: w37 -> [w139]
        tunnel: w36 -> [w138]
        stop <- w140 stop-if-true
        # "Must Delay to avoid 100% CPU"
        # "Broadcast FGGA UDP Data"
        n185 = call-poly <vilib>:"UDP Multicast Open.vi"("time-to-live (1)"=u16 5, "port"=u16 10000) -> ("error out"=w147:errorcluster, "connection ID"=w148:refnum<k16>)  [unwired: 8 in]
        n186 = node-c288() -> (w150:T1)  [unwired: 4 in]
        n187 = timed-loop {
          tunnel: w148 -> [w171]
          tunnel: w147 -> [w170]
          timing: w150 -> [_]
          timing-out: [_] -> w149
          shift-right: [w159] -> _
          shift-left: FALSE -> [w162]
          tunnel: [w158] -> w142
          tunnel: [w156] -> w141
          tunnel: [w154] -> w140
          tunnel: w139 -> [w152]
          tunnel: w138 -> [w151]
          stop <- w155 stop-if-true
          # "UDP Broadcast loop"
          n188 = node-c288() -> ()  [unwired: 1 in, 1 out]
          n189 = local read "Flight Number"() -> (w153:string)
          n190 = feedback-in #2(w153) -> ()
          n191 = feedback #2() -> (w164:string)  [unwired: 1 in]
          n192 = Not Equal?(x=w153, y=w164) -> (x != y?=w163:bool)
          n193 = String To IP(1:"239.1.4.6" ("name")) -> (0:w168:u32)
          n194 = flat-sequence {
            tunnel: w168 -> [w178]
            tunnel: w170 -> [w179]
            tunnel: w171 -> [w180]
            tunnel: [w180] -> w167
            tunnel: [w179] -> w166
            tunnel: [w178] -> w165
            tunnel: w163 -> [w177]
            tunnel: u16 50001 ("port or service name") -> [w191]
            tunnel: w167 -> [w190]
            tunnel: w166 -> [w189]
            tunnel: w165 -> [w188]
            tunnel: [w187] -> w158
            tunnel: [w186] -> w156
            tunnel: w152 -> [w184]
            tunnel: w151 -> [w183]
            frame #0 {
              n195 = feedback #3(u32 0) -> (w174:u32)
              n196 = case shown="False" w177 {
                tunnel: w174 -> [w181 _]
                tunnel: [w181 u32 0] -> w173
                frame False {
                }
                frame True {
                }
              }
              "UDP_Pack_num" <- w173
              n197 = Increment(x=w173) -> (x+1=w175:u32)
              n198 = feedback-in #3(w175) -> ()
            }
            frame #1 {
              n199 = Dequeue Element(queue=w184, error in (no error)=w183) -> (element=w185:string)  [unwired: 1 in, 3 out]
              n200 = UDP Write(address=w188, port or service name=w191, connection ID=w190, data in=w185, 8:w189) -> (error out=w186:errorcluster, 3:w187:refnum<k16>)  [unwired: 1 in]
            }
          }
          n201 = Select(t=FALSE, s=w162, f=TRUE) -> (s? t:f=w159:bool)
          "UDP_Out Status" <- w159
          n202 = local read "stop"() -> (w154:bool)
          n203 = node-c288() -> ()  [unwired: 1 in, 1 out]
          n204 = Unbundle(w156) -> ("status"=w157:bool)  [unwired: 2 out]
          n205 = Compound Arithmetic op=OR(w157, w154) -> (w155:bool)
        }
        n206 = node-c288(w149) -> ()  [unwired: 1 out]
        n207 = UDP Close(connection ID=w142, 8:w141) -> (error out=→"UDP_Out_Error Out":errorcluster)  [unwired: 1 out]
        n208 = Wait (ms)(milliseconds to wait=u32 1000) -> ()  [unwired: 1 out]
      }
      n209 = while {
        tunnel: w33 -> [w97]
        tunnel: w32 -> [w96]
        stop <- w100 stop-if-true
        # "Must Delay to avoid 100% CPU"
        # "TCP Loop writing to FISH Tank"
        n210 = TCP Open Connection(address="192.168.101.110", remote port or service name=u16 3502) -> (connection ID=w103:refnum<k5>, error out=w98:errorcluster)  [unwired: 3 in]
        n211 = case shown="No Error" w98 {
          selector: w98 -> [w108 w135]
          tunnel: w103 -> [w113 w136]
          tunnel: [w112 w136] -> w102
          tunnel: [w111 w135] -> w101
          tunnel: [w110 w134] -> w100
          tunnel: w97 -> [w107 _]
          tunnel: w96 -> [w106 _]
          frame No Error {
            n212 = node-c288() -> (w115:T1)  [unwired: 4 in]
            n213 = timed-loop {
              tunnel: w113 -> [w129]
              tunnel: w108 -> [w128]
              tunnel: [w127] -> w112
              tunnel: [w126] -> w111
              tunnel: [w118] -> w110
              shift-right: [w120] -> _
              shift-left: FALSE -> [w123]
              timing: w115 -> [_]
              timing-out: [_] -> w114
              tunnel: w107 -> [w117]
              tunnel: w106 -> [w116]
              stop <- w124 stop-if-true
              n214 = node-c288() -> ()  [unwired: 1 in, 1 out]
              n215 = Dequeue Element(queue=w117, error in (no error)=w116) -> (element=w119:string)  [unwired: 1 in, 3 out]
              n216 = Select(t=FALSE, s=w123, f=TRUE) -> (s? t:f=w120:bool)
              "TCP packet\nSend To FISH" <- w120
              n217 = TCP Write(connection ID=w129, data in=w119, error in (no error)=w128) -> (connection ID out=w127:refnum<k5>, error out=w126:errorcluster)  [unwired: 1 in, 1 out]
              n218 = local read "stop"() -> (w118:bool)
              n219 = Unbundle(w126) -> ("status"=w125:bool)  [unwired: 2 out]
              n220 = node-c288() -> ()  [unwired: 1 in, 1 out]
              n221 = Compound Arithmetic op=OR(w125, w118) -> (w124:bool)
            }
            n222 = node-c288(w114) -> ()  [unwired: 1 out]
          }
          frame Error {
            n223 = local read "stop"() -> (w134:bool)
          }
        }
        n224 = TCP Close Connection(connection ID=w102, error in (no error)=w101) -> (error out=→"FISH TCP Error Out":errorcluster)  [unwired: 1 in, 1 out]
        n225 = Wait (ms)(milliseconds to wait=u32 1000) -> ()  [unwired: 1 out]
      }
      n226 = while {
        tunnel: w35 -> [w366]
        tunnel: w34 -> [w365]
        stop <- w369 stop-if-true
        # "Must Delay to avoid 100% CPU"
        # "TCP Loop writing to SEPTIC Tank"
        n227 = TCP Open Connection(address="192.168.101.108", remote port or service name=u16 3502) -> (connection ID=w372:refnum<k5>, error out=w367:errorcluster)  [unwired: 3 in]
        n228 = case shown="No Error" w367 {
          selector: w367 -> [w377 w404]
          tunnel: w372 -> [w382 w405]
          tunnel: [w381 w405] -> w371
          tunnel: [w380 w404] -> w370
          tunnel: [w379 w403] -> w369
          tunnel: w366 -> [w376 _]
          tunnel: w365 -> [w375 _]
          frame No Error {
            n229 = node-c288() -> (w384:T1)  [unwired: 4 in]
            n230 = timed-loop {
              tunnel: w382 -> [w398]
              tunnel: w377 -> [w397]
              tunnel: [w396] -> w381
              tunnel: [w395] -> w380
              tunnel: [w387] -> w379
              shift-right: [w389] -> _
              shift-left: FALSE -> [w392]
              timing: w384 -> [_]
              timing-out: [_] -> w383
              tunnel: w376 -> [w386]
              tunnel: w375 -> [w385]
              stop <- w393 stop-if-true
              n231 = node-c288() -> ()  [unwired: 1 in, 1 out]
              n232 = Dequeue Element(queue=w386, error in (no error)=w385) -> (element=w388:string)  [unwired: 1 in, 3 out]
              n233 = Select(t=FALSE, s=w392, f=TRUE) -> (s? t:f=w389:bool)
              "TCP packet\nSend To SEPTIC" <- w389
              n234 = TCP Write(connection ID=w398, data in=w388, error in (no error)=w397) -> (connection ID out=w396:refnum<k5>, error out=w395:errorcluster)  [unwired: 1 in, 1 out]
              n235 = local read "stop"() -> (w387:bool)
              n236 = Unbundle(w395) -> ("status"=w394:bool)  [unwired: 2 out]
              n237 = node-c288() -> ()  [unwired: 1 in, 1 out]
              n238 = Compound Arithmetic op=OR(w394, w387) -> (w393:bool)
            }
            n239 = node-c288(w383) -> ()  [unwired: 1 out]
          }
          frame Error {
            n240 = local read "stop"() -> (w403:bool)
          }
        }
        n241 = TCP Close Connection(connection ID=w371, error in (no error)=w370) -> (error out=→"SEPTIC TCP Error Out":errorcluster)  [unwired: 1 in, 1 out]
        n242 = Wait (ms)(milliseconds to wait=u32 1000) -> ()  [unwired: 1 out]
      }
      n243 = node-c288(w23) -> ()  [unwired: 1 out]
    }
    frame Error {
    }
  }
  n244 = VISA Close(VISA resource name=w17, error in (no error)=w18) -> (error out=→"Serial error out":errorcluster)
